vi "Real Matrix Characteristic Polynomial.vi"(3 "A":T1) -> (0 "error":i32, 1 "Characteristic Polynomial":dbl[](array[numeric]) format="%.2f")   [LabVIEW 2017, in "NI_AALPro.lvlib"]
doc: "Calculates the characteristic polynomial of the given matrix."
uses:
  NI_AALPro.lvlib
  RealMatrix.ctl
  lvanlys.dll
  NI_Matrix.lvlib
panel:
  # "Real Matrix Characteristic Polynomial"
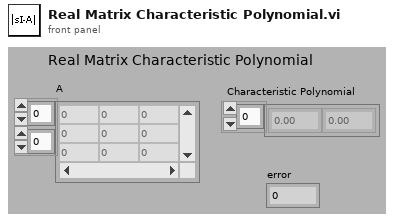
[diagram p1: front panel]
types:
  T1 = typedef "NI_Matrix.lvlib/RealMatrix.ctl" = dbl[][]
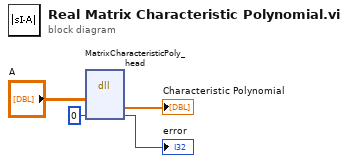
[diagram p0: block diagram]
diagram:
  n1 = dll-call lib="C:/Program Files/National Instruments/LabVIEW 2017/resource/lvanlys.*" fn="MatrixCharacteristicPoly_head"("A"="A", "error"=0) -> ("Characteristic Polynomial"=→"Characteristic Polynomial":dbl[], "error"=→"error":i32)  [unwired: 6 in, 2 out]
